vi "rqcBob SPI.Send PM Levels Values.vi"(8 "error in":errorcluster, 10 "RndGen.parameters":T1={"value type"=enum."constant", "constant"=0, "num of levels"=0, "levels values"=[0, 0, 0, 0]}, 11 "Bob FPGA Reference In":refnum<k20>) -> (0 "error out":errorcluster, 2 "Array":u32[](array[numeric]), 3 "Bob FPGA Reference Out":refnum<k20>)   [LabVIEW 2018]
uses:
  Shared/Shared FPGA Lib/Shared Logic/Custom Controls/rqc Random Generator.parameters.ctl
  Shared/Shared FPGA Lib/Shared Logic/Custom Controls/rqc Random Generator.value type.ctl
  Shared/Shared Host Lib/SPI/typedefs/SPI.FPGA Interface.ctl
  Shared/Shared Host Lib/SPI/typedefs/SPI.SubSystem.ctl
  <vilib>/Utility/error.llb/Error Cluster From Error Code.vi
  <vilib>/rvi/errors/niLvFpgaAdjustHostInterfaceError.vi
  <vilib>/rvi/interface/nirviReadWriteControl/nirviReadWriteControl.xnode
  NiFpgaLv.dll
  <vilib>/rvi/interface/Simulation/niFpgaSimulationCallBeginRW.vi
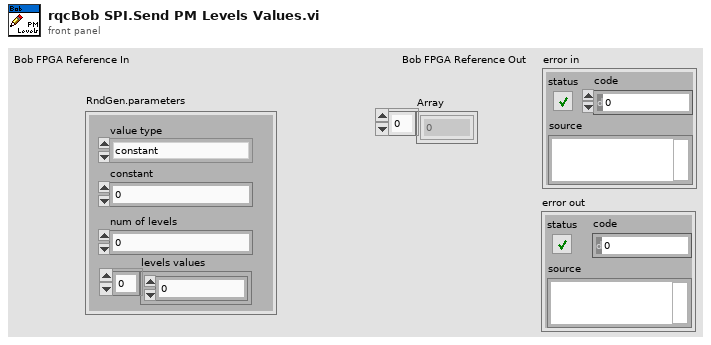
[diagram p1: front panel]
types:
  T1 = typedef "rqc Random Generator.parameters.ctl" = cluster{"value type":T2, "constant":u16, "num of levels":u16, "levels values":u16[]}
  T2 = typedef "rqc Random Generator.value type.ctl" = enum16{"random value", "constant"}
  T3 = typedef "SPI.FPGA Interface.ctl" = refnum<k20>
  T4 = typedef "SPI.SubSystem.ctl" = enum8{"N/A", "DelayLine.MSB", "DelayLine.LSB", "Attenuation.dB", "Attenuation.DAC value", "SyncDetector.Offset", "SyncDetector.Comparator", "PM.Value[0]", "PM.Value[1]", "PM.Value[2]", "PM.Value[3]"}
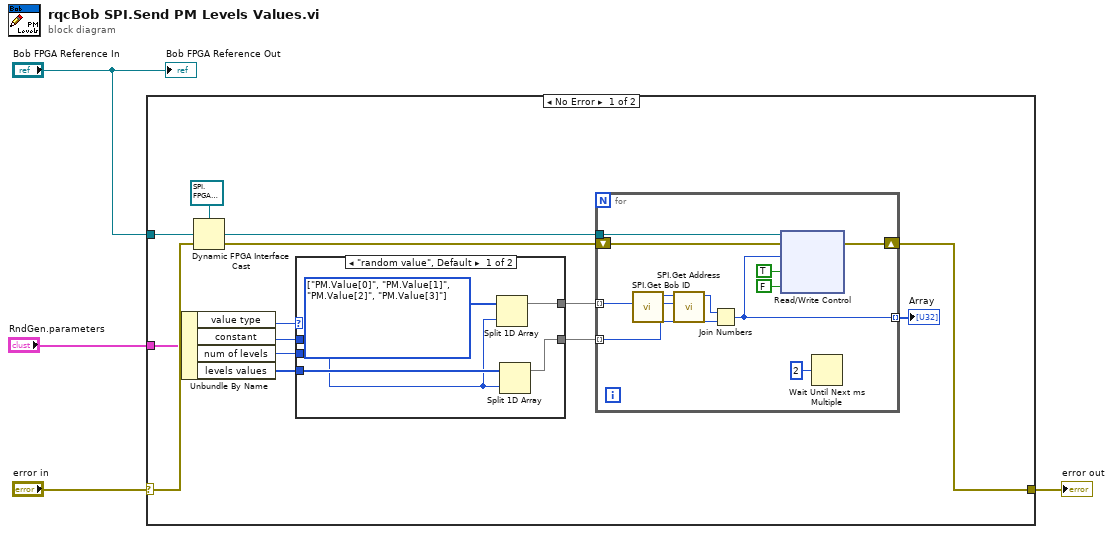
[diagram p0: block diagram]
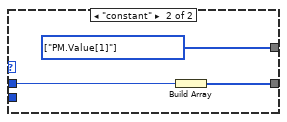
[diagram p2: hidden frame]
diagram:
  n1 = case shown="No Error" "error in" {
    selector: "error in" -> [w13 w37]
    tunnel: [w14 w37] -> w3
    tunnel: "Bob FPGA Reference In" -> [w17 _]
    tunnel: "RndGen.parameters" -> [w11 _]
    frame No Error {
      n2 = Unbundle By Name(w11) -> ("value type"=w10:T2, "constant"=w9:u16, "num of levels"=w6:u16, "levels values"=w7:u16[])
      n3 = Dynamic FPGA Interface Cast(Session In=T3 refnum ("Type"), Type=w17) -> (Session Out=w15:T3)
      n4 = case shown="\"random value\", Default" w10 {
        tunnel: [w20 w25] -> w12
        tunnel: [w18 w23] -> w8
        tunnel: w9 -> [_ w24]
        tunnel: w7 -> [w21 _]
        tunnel: w6 -> [w19 _]
        frame "random value", Default {
          w22 = T4[] [enum."PM.Value[0]", enum."PM.Value[1]", enum."PM.Value[2]", enum."PM.Value[3]"] items=["N/A", "DelayLine.MSB", "DelayLine.LSB", "Attenuation.dB", "Attenuation.DAC value", "SyncDetector.Offset", "SyncDetector.Comparator", "PM.Value[0]", "PM.Value[1]", "PM.Value[2]", "PM.Value[3]"] ("Array")
          n5 = Split 1D Array(array=w22, index=w19) -> (first subarray=w20:T4[])  [unwired: 1 out]
          n6 = Split 1D Array(array=w21, index=w19) -> (first subarray=w18:u16[])  [unwired: 1 out]
        }
        frame "constant" {
          w25 = T4[] [enum."PM.Value[1]"] items=["N/A", "DelayLine.MSB", "DelayLine.LSB", "Attenuation.dB", "Attenuation.DAC value", "SyncDetector.Offset", "SyncDetector.Comparator", "PM.Value[0]", "PM.Value[1]", "PM.Value[2]", "PM.Value[3]"] ("Array")
          n7 = Build Array(w24) -> (w23:u16[])
        }
      }
      n8 = for {
        tunnel: w15 -> [w34]
        shift-right: [w31] -> w14
        shift-left: w13 -> [w30]
        tunnel: w12 -> [w29] mode=indexing
        tunnel: w8 -> [w28] mode=indexing
        tunnel: [w26] -> w5 mode=indexing
        n9 = call "SPI.Get Bob ID.vi"() -> ("Bob.ID"=w32:u8)  [unwired: 11 in]
        n10 = call "SPI.Get Address.vi"("SPI.subSystem"=w29, "ID"=w32) -> ("Address"=w33:u16)  [unwired: 9 in]
        n11 = Join Numbers(hi=w33, lo=w28) -> ((hi.lo)=w26:u32)
        n12 = xnode "Read/Write Control"("FPGA VI Reference In"=w34, "error in"=w30, "SPI.data"=w26, "SPI.write"=TRUE ("reset"), "SPI.write"=FALSE ("reset")) -> ("error out"=w31:errorcluster)  [unwired: 1 out]
        n13 = Wait Until Next ms Multiple(millisecond multiple=u32 2) -> ()  [unwired: 1 out]
      }
      "Array" <- w5
    }
    frame Error {
    }
  }
  "error out" <- w3
  "Bob FPGA Reference Out" <- "Bob FPGA Reference In"
